vi "Conection List.vi"(0 "ModbusSp in":refnum<class "ModbusSp.lvclass">, 11 "error in (no error)":errorcluster) -> (4 "ModbusSp out":refnum<class "ModbusSp.lvclass">, 6 "TCP Connection Count":u32, 8 "TCP Connection List":T1[](array[typedef]), 15 "error out":errorcluster)   [LabVIEW 2019, in "ModbusSp.lvclass"]
uses:
  ModbusSp.lvclass
  <vilib>/NI/Modbus Library/Network Protocol/Network Slave/TCP/Connection.ctl
  ModbusSp.lvclass/ModbusSp.ctl
  <vilib>/NI/Modbus Library/API/Slave/Modbus Slave.lvclass
  <vilib>/NI/Modbus Library/Network Protocol/Network Slave/TCP/TCP Slave.lvclass
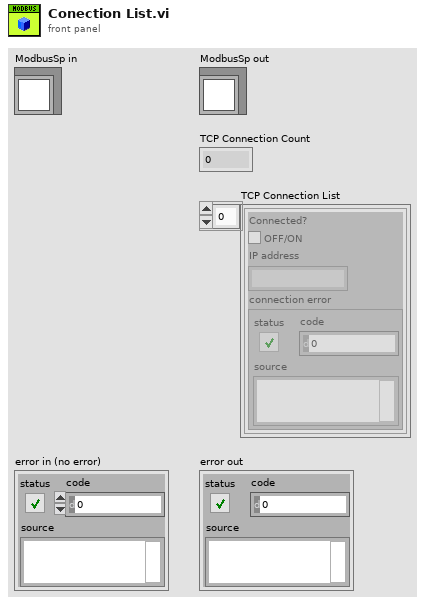
[diagram p1: front panel]
types:
  T1 = typedef "TCP Slave.lvclass/Connection.ctl" = cluster{"Connected?":bool, "IP address":string, "connection error":errorcluster}
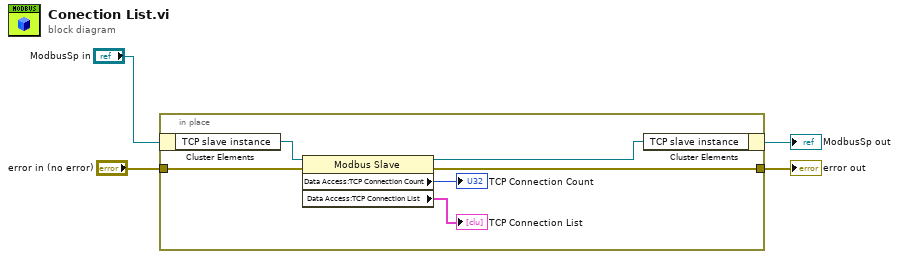
[diagram p0: block diagram]
diagram:
  n1 = in-place {
    in-place-border: [w7] -> w3
    in-place-border: "error in (no error)" -> [w9]
    n2 = in-place-cluster #1("ModbusSp in") -> ("TCP slave instance"=w10:refnum<class "Modbus Slave.lvclass">)
    n3 = property class="Modbus Slave"(reference=w10, error in=w9) -> (reference out=w8:refnum<class "Modbus Slave.lvclass">, error out=w7:errorcluster, "Data Access:TCP Connection Count"=→"TCP Connection Count":u32, "Data Access:TCP Connection List"=→"TCP Connection List":T1[])
    n4 = in-place-cluster #1("TCP slave instance"=w8) -> (→"ModbusSp out":refnum<class "ModbusSp.lvclass">)
  }
  "error out" <- w3
